vi "compass.vi"(4 "center":cluster{"x":i32, "y":i32}={"x"=38, "y"=38}, 6 "size":i16=32, 7 "angle":i32(slide)=4 scale=-360.0..360.0, 10 "pict in":picture) -> (3 "pict out":picture)   [LabVIEW 2011]
panel:
  in  "average_angle":i32
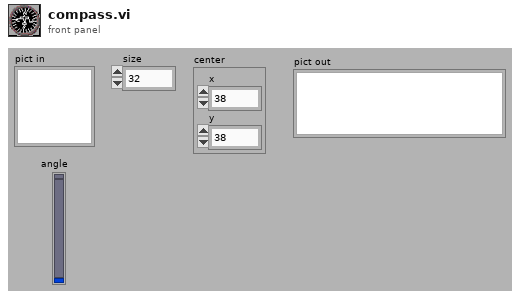
[diagram p1: front panel]
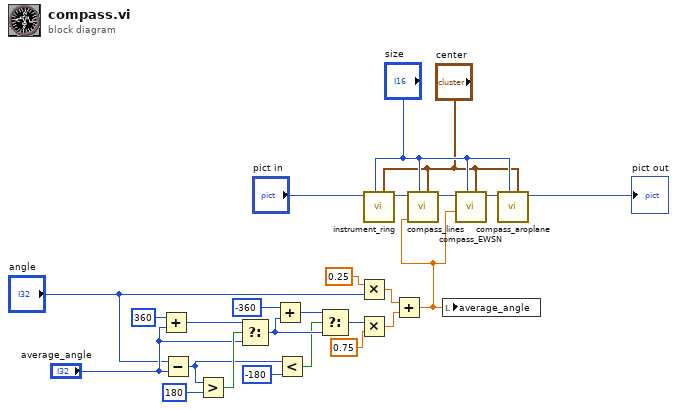
[diagram p0: block diagram]
diagram:
  n1 = Add(x=360, y="average_angle") -> (x+y=w14:i32)
  n2 = Subtract(x="angle", y="average_angle") -> (x-y=w11:i32)
  n3 = Greater?(x=w11, y=180) -> (0:w12:bool)
  n4 = Select(t=w14, s=w12, f="average_angle") -> (s? t:f=w9:i32)
  n5 = Add(x=-360, y=w9) -> (x+y=w7:i32)
  n6 = Less?(x=w11, y=-180) -> (x < y?=w6:bool)
  n7 = Select(t=w7, s=w6, f=w9) -> (s? t:f=w3:i32)
  n8 = Multiply(x=0.25, y="angle") -> (x*y=w16:dbl)
  n9 = Multiply(x=w3, y=0.75) -> (x*y=w4:dbl)
  n10 = call "instrument_ring.vi"("center"="center", "size"="size", "pict in"="pict in") -> ("new picture"=w20:picture)  [unwired: 7 in]
  n11 = Add(x=w16, y=w4) -> (x+y=w2:dbl)
  n12 = call "compass_lines.vi"("center"="center", "size"="size", "angle"=w2, "pict in"=w20) -> ("pict out"=w21:picture)  [unwired: 6 in]
  n13 = local write "average_angle"(w2) -> ()
  n14 = call "compass_EWSN.vi"("center"="center", "size"="size", "angle"=w2, "pict in"=w21) -> ("pict out"=w22:picture)  [unwired: 6 in]
  n15 = call "compass_aroplane.vi"("center"="center", "size"="size", "pict in"=w22) -> ("pict out"=→"pict out":picture)  [unwired: 7 in]
